vi "LEP_RV_Error.vi"(8 "Message(s)":string, 11 "title":string) -> ()   [LabVIEW 2011]
doc: "Displays <B>Error Message</B> and <B>Error Output</B> in the <B>Failed to build executable</B> dialog box."
panel:
  in  "ok":bool
  out "Detailed Output":string
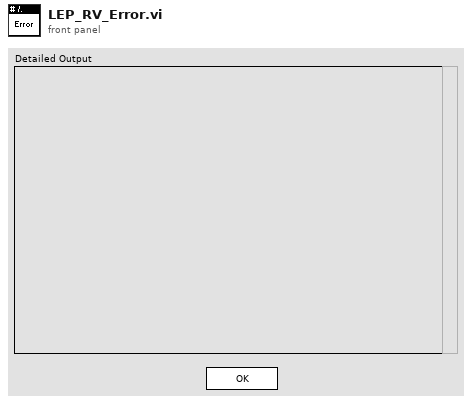
[diagram p1: front panel]
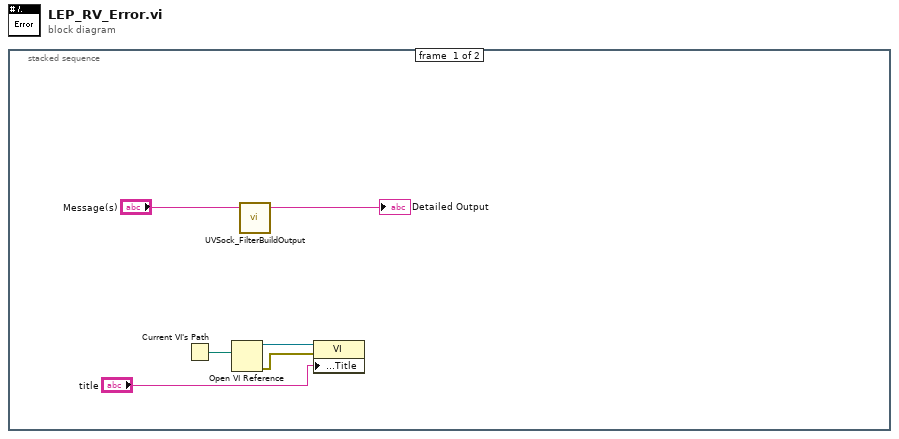
[diagram p0: block diagram]
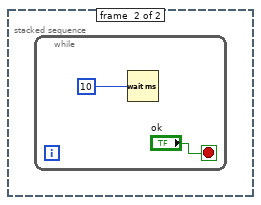
[diagram p2: hidden frame]
diagram:
  n1 = stacked-sequence {
    frame #0 {
      n2 = Current VI's Path() -> (path=w6:path)
      n3 = Open VI Reference(vi path=w6) -> (vi reference=w5:refnum<vi>, error out=w4:errorcluster)  [unwired: 5 in]
      n4 = call "UVSock_FilterBuildOutput.vi"("build output"="Message(s)") -> ("filtered build output"=→"Detailed Output":string)  [unwired: 3 in, 1 out]
      n5 = property class="VI"(reference=w5, error in=w4, "Front Panel.Title"="title") -> ()  [unwired: 2 out]
    }
    frame #1 {
      n6 = while {
        stop <- "ok" stop-if-true
        n7 = Wait (ms)(milliseconds to wait=u32 10) -> ()  [unwired: 1 out]
      }
    }
  }
